vi "Calculate 2D scan positions.vi"(2 "Scan direction":u16(ring) items=["Scan from middle", "Scan upper left", "Scan upper right", "Scan lower left", "Scan lower right", "Scan left", "Scan right", "Scan above", "Scan below"], 3 "Start position ax1":dbl format="%.6f", 4 "Start position ax2":dbl format="%.6f", 6 "Range ax1":dbl format="%.2f", 7 "Step size ax1":dbl format="%.2f", 8 "Range ax2":dbl format="%.2f", 9 "Step size ax2":dbl format="%.2f") -> (10 "Min. pos. ax2":dbl format="%.6f", 11 "Max. pos. ax2":dbl format="%.6f", 12 "1D pos. array ax2":dbl[](array[numeric]) format="%.6f", 13 "No. of steps ax2":i32, 14 "1D pos. array ax1":dbl[](array[numeric]) format="%.6f", 15 "Min. pos. ax1":dbl format="%.6f", 16 "Max. pos. ax1":dbl format="%.6f", 17 "No. of steps ax1":i32, 18 "2D intensity array":dbl[][](array[numeric]) format="%.6f")   [LabVIEW 2020]
doc: "Calculates 2D scan positions according to Scan direction, Start position, Range and Step size of axes 1 and 2 and returns Minimum position, Maximum position, No. of steps and initialized 1D position array for axes 1 and 2 and a 2D intensity array. Scan direction can be \n- Scan from middle meaning that the scan starts at (Start position ax1 - ½ Range ax1, Start position ax2 - ½ Range ax2) and stops at (Start position ax1 + ½ Range ax1, Start position ax2 + ½ Range ax2), \n- Scan upper left meaning that scan starts at (Start position ax1 - Range ax1, Start position ax2) and stops at (Start position ax1, Start position ax2 + Range ax2), \n- Scan upper right meaning that scan starts at (Start position ax1, Start position ax2) and stops at (Start position ax1 + Range ax1, Start position ax2 + Range ax2), \n- Scan lower left meaning that the scan starts at (Start position ax1 - Range ax1, Start position ax2 - Range ax2) and stops at (Start position ax1, Start position ax2), \n- Scan lower right meaning that the scan starts at (Start position ax1, Start position ax2 - Range ax2) and stops at (Start position ax1 + Range ax1, Start position ax2), \n- Scan left meaning that the scan starts at (Start position ax1 - Range ax1, Start position ax2 - ½ Range ax2) and stops at (Start position ax1, Start position ax2 + ½ Range ax2), \n- Scan right meaning that the scan starts at (Start position ax1, Start position ax2 - ½ Range ax2) and stops at (Start position ax1 + Range ax1, Start position ax2 + ½ Range ax2), \n- Scan above meaning that the scan starts at (Start position ax1 - ½ Range ax1, Start position ax2) and stops at (Start position ax1 + ½ Range ax1, Start position ax2 + Range ax2), \n- Scan below meaning that the scan starts at (Start position ax1 - ½ Range ax1, Start position ax2 - Range ax2) and stops at (Start position ax1 + ½ Range ax1, Start position ax2),"
panel:
  # "Calculates 2D scan positions and initialized intensity array."
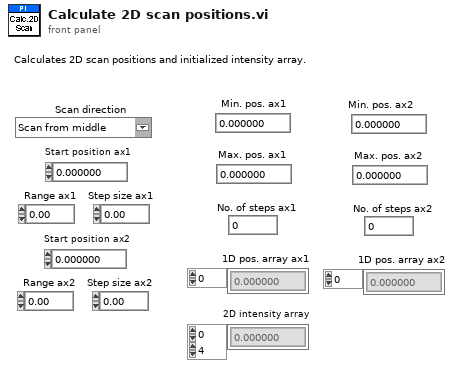
[diagram p1: front panel]
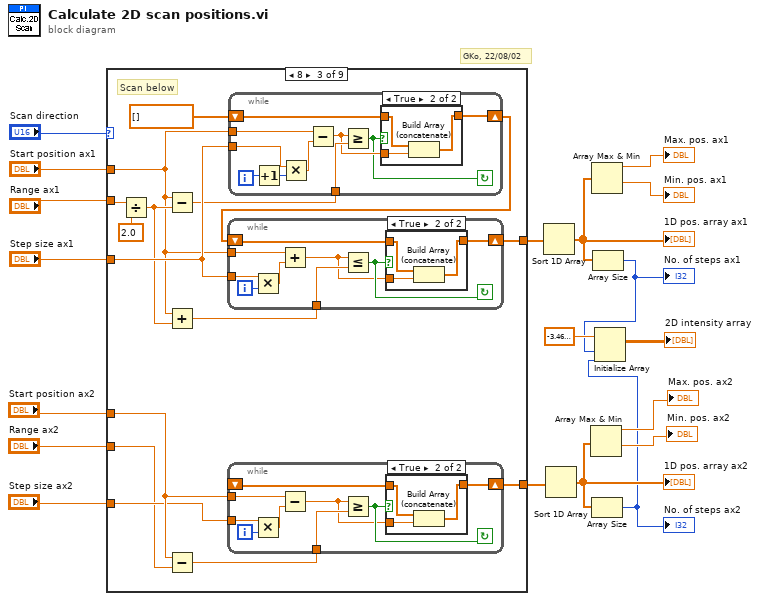
[diagram p0: block diagram]
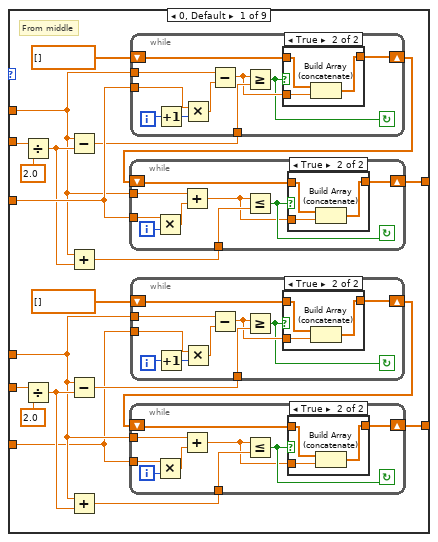
[diagram p2: hidden frame]
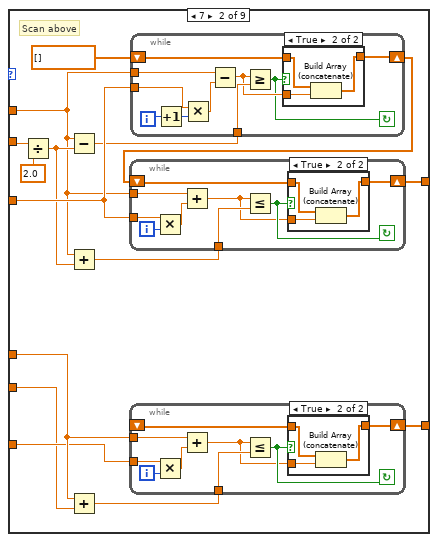
[diagram p7: hidden frame]
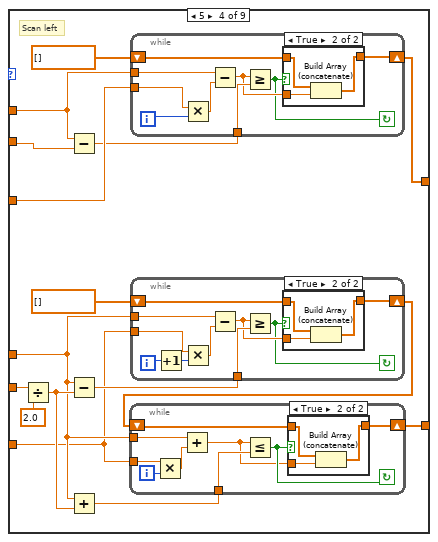
[diagram p14: hidden frame]
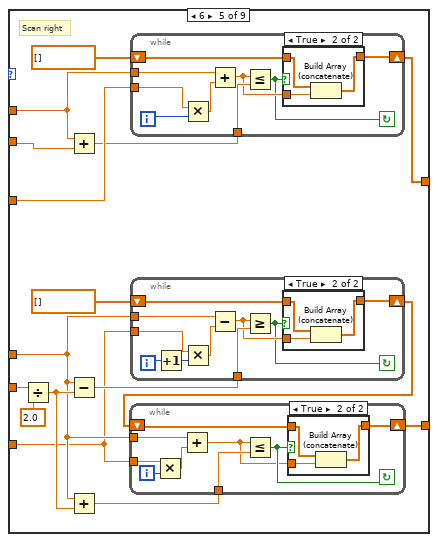
[diagram p18: hidden frame]
diagram:
  # "GKo, 22/08/02"
  n1 = case shown="8" "Scan direction" {
    tunnel: "Range ax1" -> [w39 w108 w163 w204 w260 w325 w363 w401 w439]
    tunnel: "Start position ax1" -> [w34 w103 w158 w218 w274 w326 w364 w402 w440]
    tunnel: "Step size ax1" -> [w36 w105 w160 w219 w275 w327 w365 w403 w441]
    tunnel: [w30 w99 w154 w205 w261 w322 w360 w398 w436] -> w11
    tunnel: [w23 w97 w152 w209 w265 w319 w357 w395 w433] -> w9
    tunnel: "Range ax2" -> [w22 w94 w149 w208 w264 w317 w355 w393 w431]
    tunnel: "Start position ax2" -> [w21 w96 w151 w207 w263 w318 w356 w394 w432]
    tunnel: "Step size ax2" -> [w20 w95 w150 w206 w262 w316 w354 w392 w430]
    frame 0, Default {
      # "From middle"
      n2 = Divide(x=w39, y=2.0) -> (x/y=w35:dbl)
      n3 = Divide(x=w22, y=2.0) -> (x/y=w27:dbl)
      n4 = Subtract(x=w34, y=w35) -> (x-y=w33:dbl)
      n5 = Add(x=w34, y=w35) -> (x+y=w37:dbl)
      n6 = Subtract(x=w21, y=w27) -> (x-y=w26:dbl)
      n7 = Add(x=w21, y=w27) -> (x+y=w28:dbl)
      n8 = while {
        shift-left: dbl[] [] -> [w56]
        shift-right: [w54] -> w31
        tunnel: w33 -> [w57]
        tunnel: w36 -> [w59]
        tunnel: w34 -> [w61]
        i -> [w62]
        stop <- w53 continue-if-true
        n9 = Increment(x=w62) -> (x+1=w60:i32)
        n10 = Multiply(x=w59, y=w60) -> (x*y=w58:dbl)
        n11 = Subtract(x=w61, y=w58) -> (x-y=w55:dbl)
        n12 = Greater Or Equal?(x=w55, y=w57) -> (x >= y?=w53:bool)
        n13 = case shown="True" w53 {
          tunnel: [w63 w66] -> w54
          tunnel: w56 -> [w63 w65]
          tunnel: w55 -> [_ w64]
          frame False {
          }
          frame True {
            n14 = Build Array (concatenate)(w65, w64) -> (w66:dbl[])
          }
        }
      }
      n15 = while {
        tunnel: w37 -> [w42]
        shift-left: w31 -> [w43]
        shift-right: [w44] -> w30
        tunnel: w34 -> [w46]
        tunnel: w36 -> [w47]
        i -> [w48]
        stop <- w41 continue-if-true
        n16 = Multiply(x=w47, y=w48) -> (x*y=w45:dbl)
        n17 = Add(x=w46, y=w45) -> (x+y=w40:dbl)
        n18 = Less Or Equal?(x=w40, y=w42) -> (x <= y?=w41:bool)
        n19 = case shown="True" w41 {
          tunnel: [w49 w52] -> w44
          tunnel: w43 -> [w49 w51]
          tunnel: w40 -> [_ w50]
          frame False {
          }
          frame True {
            n20 = Build Array (concatenate)(w51, w50) -> (w52:dbl[])
          }
        }
      }
      n21 = while {
        shift-left: dbl[] [] -> [w83]
        shift-right: [w81] -> w24
        tunnel: w26 -> [w84]
        tunnel: w20 -> [w86]
        tunnel: w21 -> [w88]
        i -> [w89]
        stop <- w80 continue-if-true
        n22 = Increment(x=w89) -> (x+1=w87:i32)
        n23 = Multiply(x=w86, y=w87) -> (x*y=w85:dbl)
        n24 = Subtract(x=w88, y=w85) -> (x-y=w82:dbl)
        n25 = Greater Or Equal?(x=w82, y=w84) -> (x >= y?=w80:bool)
        n26 = case shown="True" w80 {
          tunnel: [w90 w93] -> w81
          tunnel: w83 -> [w90 w92]
          tunnel: w82 -> [_ w91]
          frame False {
          }
          frame True {
            n27 = Build Array (concatenate)(w92, w91) -> (w93:dbl[])
          }
        }
      }
      n28 = while {
        tunnel: w28 -> [w69]
        shift-left: w24 -> [w70]
        shift-right: [w71] -> w23
        tunnel: w21 -> [w73]
        tunnel: w20 -> [w74]
        i -> [w75]
        stop <- w68 continue-if-true
        n29 = Multiply(x=w74, y=w75) -> (x*y=w72:dbl)
        n30 = Add(x=w73, y=w72) -> (x+y=w67:dbl)
        n31 = Less Or Equal?(x=w67, y=w69) -> (x <= y?=w68:bool)
        n32 = case shown="True" w68 {
          tunnel: [w76 w79] -> w71
          tunnel: w70 -> [w76 w78]
          tunnel: w67 -> [_ w77]
          frame False {
          }
          frame True {
            n33 = Build Array (concatenate)(w78, w77) -> (w79:dbl[])
          }
        }
      }
    }
    frame 7 {
      # "Scan above"
      n34 = Divide(x=w108, y=2.0) -> (x/y=w104:dbl)
      n35 = Subtract(x=w103, y=w104) -> (x-y=w102:dbl)
      n36 = Add(x=w103, y=w104) -> (x+y=w106:dbl)
      n37 = Add(x=w96, y=w94) -> (x+y=w98:dbl)
      n38 = while {
        tunnel: w98 -> [w138]
        shift-left: _ -> [w139]
        shift-right: [w140] -> w97
        tunnel: w96 -> [w142]
        tunnel: w95 -> [w143]
        i -> [w144]
        stop <- w137 continue-if-true
        n39 = Multiply(x=w143, y=w144) -> (x*y=w141:dbl)
        n40 = Add(x=w142, y=w141) -> (x+y=w136:dbl)
        n41 = Less Or Equal?(x=w136, y=w138) -> (x <= y?=w137:bool)
        n42 = case shown="True" w137 {
          tunnel: [w145 w148] -> w140
          tunnel: w139 -> [w145 w147]
          tunnel: w136 -> [_ w146]
          frame False {
          }
          frame True {
            n43 = Build Array (concatenate)(w147, w146) -> (w148:dbl[])
          }
        }
      }
      n44 = while {
        shift-left: dbl[] [] -> [w125]
        shift-right: [w123] -> w100
        tunnel: w102 -> [w126]
        tunnel: w105 -> [w128]
        tunnel: w103 -> [w130]
        i -> [w131]
        stop <- w122 continue-if-true
        n45 = Increment(x=w131) -> (x+1=w129:i32)
        n46 = Multiply(x=w128, y=w129) -> (x*y=w127:dbl)
        n47 = Subtract(x=w130, y=w127) -> (x-y=w124:dbl)
        n48 = Greater Or Equal?(x=w124, y=w126) -> (x >= y?=w122:bool)
        n49 = case shown="True" w122 {
          tunnel: [w132 w135] -> w123
          tunnel: w125 -> [w132 w134]
          tunnel: w124 -> [_ w133]
          frame False {
          }
          frame True {
            n50 = Build Array (concatenate)(w134, w133) -> (w135:dbl[])
          }
        }
      }
      n51 = while {
        tunnel: w106 -> [w111]
        shift-left: w100 -> [w112]
        shift-right: [w113] -> w99
        tunnel: w103 -> [w115]
        tunnel: w105 -> [w116]
        i -> [w117]
        stop <- w110 continue-if-true
        n52 = Multiply(x=w116, y=w117) -> (x*y=w114:dbl)
        n53 = Add(x=w115, y=w114) -> (x+y=w109:dbl)
        n54 = Less Or Equal?(x=w109, y=w111) -> (x <= y?=w110:bool)
        n55 = case shown="True" w110 {
          tunnel: [w118 w121] -> w113
          tunnel: w112 -> [w118 w120]
          tunnel: w109 -> [_ w119]
          frame False {
          }
          frame True {
            n56 = Build Array (concatenate)(w120, w119) -> (w121:dbl[])
          }
        }
      }
    }
    frame 8 {
      # "Scan below"
      n57 = Divide(x=w163, y=2.0) -> (x/y=w159:dbl)
      n58 = Subtract(x=w158, y=w159) -> (x-y=w157:dbl)
      n59 = Add(x=w158, y=w159) -> (x+y=w161:dbl)
      n60 = Subtract(x=w151, y=w149) -> (x-y=w153:dbl)
      n61 = while {
        tunnel: w153 -> [w193]
        shift-left: _ -> [w194]
        shift-right: [w195] -> w152
        tunnel: w151 -> [w197]
        tunnel: w150 -> [w198]
        i -> [w199]
        stop <- w192 continue-if-true
        n62 = Multiply(x=w198, y=w199) -> (x*y=w196:dbl)
        n63 = Subtract(x=w197, y=w196) -> (x-y=w191:dbl)
        n64 = Greater Or Equal?(x=w191, y=w193) -> (x >= y?=w192:bool)
        n65 = case shown="True" w192 {
          tunnel: [w200 w203] -> w195
          tunnel: w194 -> [w200 w202]
          tunnel: w191 -> [_ w201]
          frame False {
          }
          frame True {
            n66 = Build Array (concatenate)(w202, w201) -> (w203:dbl[])
          }
        }
      }
      n67 = while {
        shift-left: dbl[] [] -> [w180]
        shift-right: [w178] -> w155
        tunnel: w157 -> [w181]
        tunnel: w160 -> [w183]
        tunnel: w158 -> [w185]
        i -> [w186]
        stop <- w177 continue-if-true
        n68 = Increment(x=w186) -> (x+1=w184:i32)
        n69 = Multiply(x=w183, y=w184) -> (x*y=w182:dbl)
        n70 = Subtract(x=w185, y=w182) -> (x-y=w179:dbl)
        n71 = Greater Or Equal?(x=w179, y=w181) -> (x >= y?=w177:bool)
        n72 = case shown="True" w177 {
          tunnel: [w187 w190] -> w178
          tunnel: w180 -> [w187 w189]
          tunnel: w179 -> [_ w188]
          frame False {
          }
          frame True {
            n73 = Build Array (concatenate)(w189, w188) -> (w190:dbl[])
          }
        }
      }
      n74 = while {
        tunnel: w161 -> [w166]
        shift-left: w155 -> [w167]
        shift-right: [w168] -> w154
        tunnel: w158 -> [w170]
        tunnel: w160 -> [w171]
        i -> [w172]
        stop <- w165 continue-if-true
        n75 = Multiply(x=w171, y=w172) -> (x*y=w169:dbl)
        n76 = Add(x=w170, y=w169) -> (x+y=w164:dbl)
        n77 = Less Or Equal?(x=w164, y=w166) -> (x <= y?=w165:bool)
        n78 = case shown="True" w165 {
          tunnel: [w173 w176] -> w168
          tunnel: w167 -> [w173 w175]
          tunnel: w164 -> [_ w174]
          frame False {
          }
          frame True {
            n79 = Build Array (concatenate)(w175, w174) -> (w176:dbl[])
          }
        }
      }
    }
    frame 5 {
      # "Scan left"
      n80 = Divide(x=w208, y=2.0) -> (x/y=w213:dbl)
      n81 = Subtract(x=w218, y=w204) -> (x-y=w217:dbl)
      n82 = Subtract(x=w207, y=w213) -> (x-y=w212:dbl)
      n83 = Add(x=w207, y=w213) -> (x+y=w214:dbl)
      n84 = while {
        shift-left: dbl[] [] -> [w224]
        shift-right: [w222] -> w205
        tunnel: w217 -> [w225]
        tunnel: w219 -> [w227]
        tunnel: w218 -> [w228]
        i -> [w220]
        stop <- w221 continue-if-true
        n85 = Multiply(x=w227, y=w220) -> (x*y=w226:dbl)
        n86 = Subtract(x=w228, y=w226) -> (x-y=w223:dbl)
        n87 = Greater Or Equal?(x=w223, y=w225) -> (x >= y?=w221:bool)
        n88 = case shown="True" w221 {
          tunnel: [w229 w232] -> w222
          tunnel: w224 -> [w229 w231]
          tunnel: w223 -> [_ w230]
          frame False {
          }
          frame True {
            n89 = Build Array (concatenate)(w231, w230) -> (w232:dbl[])
          }
        }
      }
      n90 = while {
        shift-left: dbl[] [] -> [w249]
        shift-right: [w247] -> w210
        tunnel: w212 -> [w250]
        tunnel: w206 -> [w252]
        tunnel: w207 -> [w254]
        i -> [w255]
        stop <- w246 continue-if-true
        n91 = Increment(x=w255) -> (x+1=w253:i32)
        n92 = Multiply(x=w252, y=w253) -> (x*y=w251:dbl)
        n93 = Subtract(x=w254, y=w251) -> (x-y=w248:dbl)
        n94 = Greater Or Equal?(x=w248, y=w250) -> (x >= y?=w246:bool)
        n95 = case shown="True" w246 {
          tunnel: [w256 w259] -> w247
          tunnel: w249 -> [w256 w258]
          tunnel: w248 -> [_ w257]
          frame False {
          }
          frame True {
            n96 = Build Array (concatenate)(w258, w257) -> (w259:dbl[])
          }
        }
      }
      n97 = while {
        tunnel: w214 -> [w235]
        shift-left: w210 -> [w236]
        shift-right: [w237] -> w209
        tunnel: w207 -> [w239]
        tunnel: w206 -> [w240]
        i -> [w241]
        stop <- w234 continue-if-true
        n98 = Multiply(x=w240, y=w241) -> (x*y=w238:dbl)
        n99 = Add(x=w239, y=w238) -> (x+y=w233:dbl)
        n100 = Less Or Equal?(x=w233, y=w235) -> (x <= y?=w234:bool)
        n101 = case shown="True" w234 {
          tunnel: [w242 w245] -> w237
          tunnel: w236 -> [w242 w244]
          tunnel: w233 -> [_ w243]
          frame False {
          }
          frame True {
            n102 = Build Array (concatenate)(w244, w243) -> (w245:dbl[])
          }
        }
      }
    }
    frame 6 {
      # "Scan right"
      n103 = Divide(x=w264, y=2.0) -> (x/y=w269:dbl)
      n104 = Add(x=w274, y=w260) -> (x+y=w273:dbl)
      n105 = Subtract(x=w263, y=w269) -> (x-y=w268:dbl)
      n106 = Add(x=w263, y=w269) -> (x+y=w270:dbl)
      n107 = while {
        shift-left: dbl[] [] -> [w280]
        shift-right: [w278] -> w261
        tunnel: w273 -> [w281]
        tunnel: w275 -> [w283]
        tunnel: w274 -> [w284]
        i -> [w276]
        stop <- w277 continue-if-true
        n108 = Multiply(x=w283, y=w276) -> (x*y=w282:dbl)
        n109 = Add(x=w284, y=w282) -> (x+y=w279:dbl)
        n110 = Less Or Equal?(x=w279, y=w281) -> (x <= y?=w277:bool)
        n111 = case shown="True" w277 {
          tunnel: [w285 w288] -> w278
          tunnel: w280 -> [w285 w287]
          tunnel: w279 -> [_ w286]
          frame False {
          }
          frame True {
            n112 = Build Array (concatenate)(w287, w286) -> (w288:dbl[])
          }
        }
      }
      n113 = while {
        shift-left: dbl[] [] -> [w305]
        shift-right: [w303] -> w266
        tunnel: w268 -> [w306]
        tunnel: w262 -> [w308]
        tunnel: w263 -> [w310]
        i -> [w311]
        stop <- w302 continue-if-true
        n114 = Increment(x=w311) -> (x+1=w309:i32)
        n115 = Multiply(x=w308, y=w309) -> (x*y=w307:dbl)
        n116 = Subtract(x=w310, y=w307) -> (x-y=w304:dbl)
        n117 = Greater Or Equal?(x=w304, y=w306) -> (x >= y?=w302:bool)
        n118 = case shown="True" w302 {
          tunnel: [w312 w315] -> w303
          tunnel: w305 -> [w312 w314]
          tunnel: w304 -> [_ w313]
          frame False {
          }
          frame True {
            n119 = Build Array (concatenate)(w314, w313) -> (w315:dbl[])
          }
        }
      }
      n120 = while {
        tunnel: w270 -> [w291]
        shift-left: w266 -> [w292]
        shift-right: [w293] -> w265
        tunnel: w263 -> [w295]
        tunnel: w262 -> [w296]
        i -> [w297]
        stop <- w290 continue-if-true
        n121 = Multiply(x=w296, y=w297) -> (x*y=w294:dbl)
        n122 = Add(x=w295, y=w294) -> (x+y=w289:dbl)
        n123 = Less Or Equal?(x=w289, y=w291) -> (x <= y?=w290:bool)
        n124 = case shown="True" w290 {
          tunnel: [w298 w301] -> w293
          tunnel: w292 -> [w298 w300]
          tunnel: w289 -> [_ w299]
          frame False {
          }
          frame True {
            n125 = Build Array (concatenate)(w300, w299) -> (w301:dbl[])
          }
        }
      }
    }
    frame 1 {
      # "Scan upper left"
      n126 = Subtract(x=w326, y=w325) -> (x-y=w324:dbl)
      n127 = Add(x=w318, y=w317) -> (x+y=w321:dbl)
      n128 = while {
        tunnel: w324 -> [w328]
        shift-left: dbl[] [] -> [w332]
        shift-right: [w331] -> w322
        tunnel: w327 -> [w334]
        tunnel: w326 -> [w336]
        i -> [w335]
        stop <- w330 continue-if-true
        n129 = Multiply(x=w334, y=w335) -> (x*y=w333:dbl)
        n130 = Subtract(x=w336, y=w333) -> (x-y=w329:dbl)
        n131 = Greater Or Equal?(x=w329, y=w328) -> (x >= y?=w330:bool)
        n132 = case shown="True" w330 {
          tunnel: [w337 w340] -> w331
          tunnel: w332 -> [w337 w339]
          tunnel: w329 -> [_ w338]
          frame False {
          }
          frame True {
            n133 = Build Array (concatenate)(w339, w338) -> (w340:dbl[])
          }
        }
      }
      n134 = while {
        tunnel: w321 -> [w341]
        shift-left: dbl[] [] -> [w345]
        shift-right: [w344] -> w319
        tunnel: w316 -> [w347]
        tunnel: w318 -> [w349]
        i -> [w348]
        stop <- w343 continue-if-true
        n135 = Multiply(x=w347, y=w348) -> (x*y=w346:dbl)
        n136 = Add(x=w349, y=w346) -> (x+y=w342:dbl)
        n137 = Less Or Equal?(x=w342, y=w341) -> (x <= y?=w343:bool)
        n138 = case shown="True" w343 {
          tunnel: [w350 w353] -> w344
          tunnel: w345 -> [w350 w352]
          tunnel: w342 -> [_ w351]
          frame False {
          }
          frame True {
            n139 = Build Array (concatenate)(w352, w351) -> (w353:dbl[])
          }
        }
      }
    }
    frame 2 {
      # "Scan upper right"
      n140 = Add(x=w364, y=w363) -> (x+y=w362:dbl)
      n141 = Add(x=w356, y=w355) -> (x+y=w359:dbl)
      n142 = while {
        tunnel: w362 -> [w366]
        shift-left: dbl[] [] -> [w370]
        shift-right: [w369] -> w360
        tunnel: w365 -> [w372]
        tunnel: w364 -> [w374]
        i -> [w373]
        stop <- w368 continue-if-true
        n143 = Multiply(x=w372, y=w373) -> (x*y=w371:dbl)
        n144 = Add(x=w374, y=w371) -> (x+y=w367:dbl)
        n145 = Less Or Equal?(x=w367, y=w366) -> (x <= y?=w368:bool)
        n146 = case shown="True" w368 {
          tunnel: [w375 w378] -> w369
          tunnel: w370 -> [w375 w377]
          tunnel: w367 -> [_ w376]
          frame False {
          }
          frame True {
            n147 = Build Array (concatenate)(w377, w376) -> (w378:dbl[])
          }
        }
      }
      n148 = while {
        tunnel: w359 -> [w379]
        shift-left: dbl[] [] -> [w383]
        shift-right: [w382] -> w357
        tunnel: w354 -> [w385]
        tunnel: w356 -> [w387]
        i -> [w386]
        stop <- w381 continue-if-true
        n149 = Multiply(x=w385, y=w386) -> (x*y=w384:dbl)
        n150 = Add(x=w387, y=w384) -> (x+y=w380:dbl)
        n151 = Less Or Equal?(x=w380, y=w379) -> (x <= y?=w381:bool)
        n152 = case shown="True" w381 {
          tunnel: [w388 w391] -> w382
          tunnel: w383 -> [w388 w390]
          tunnel: w380 -> [_ w389]
          frame False {
          }
          frame True {
            n153 = Build Array (concatenate)(w390, w389) -> (w391:dbl[])
          }
        }
      }
    }
    frame 3 {
      # "Scan lower left"
      n154 = Subtract(x=w402, y=w401) -> (x-y=w400:dbl)
      n155 = Subtract(x=w394, y=w393) -> (x-y=w397:dbl)
      n156 = while {
        tunnel: w400 -> [w404]
        shift-left: dbl[] [] -> [w408]
        shift-right: [w407] -> w398
        tunnel: w403 -> [w410]
        tunnel: w402 -> [w412]
        i -> [w411]
        stop <- w406 continue-if-true
        n157 = Multiply(x=w410, y=w411) -> (x*y=w409:dbl)
        n158 = Subtract(x=w412, y=w409) -> (x-y=w405:dbl)
        n159 = Greater Or Equal?(x=w405, y=w404) -> (x >= y?=w406:bool)
        n160 = case shown="True" w406 {
          tunnel: [w413 w416] -> w407
          tunnel: w408 -> [w413 w415]
          tunnel: w405 -> [_ w414]
          frame False {
          }
          frame True {
            n161 = Build Array (concatenate)(w415, w414) -> (w416:dbl[])
          }
        }
      }
      n162 = while {
        tunnel: w397 -> [w417]
        shift-left: dbl[] [] -> [w421]
        shift-right: [w420] -> w395
        tunnel: w392 -> [w423]
        tunnel: w394 -> [w425]
        i -> [w424]
        stop <- w419 continue-if-true
        n163 = Multiply(x=w423, y=w424) -> (x*y=w422:dbl)
        n164 = Subtract(x=w425, y=w422) -> (x-y=w418:dbl)
        n165 = Greater Or Equal?(x=w418, y=w417) -> (x >= y?=w419:bool)
        n166 = case shown="True" w419 {
          tunnel: [w426 w429] -> w420
          tunnel: w421 -> [w426 w428]
          tunnel: w418 -> [_ w427]
          frame False {
          }
          frame True {
            n167 = Build Array (concatenate)(w428, w427) -> (w429:dbl[])
          }
        }
      }
    }
    frame 4 {
      # "Scan lower right"
      n168 = Add(x=w440, y=w439) -> (x+y=w438:dbl)
      n169 = Subtract(x=w432, y=w431) -> (x-y=w435:dbl)
      n170 = while {
        tunnel: w438 -> [w442]
        shift-left: dbl[] [] -> [w446]
        shift-right: [w445] -> w436
        tunnel: w441 -> [w448]
        tunnel: w440 -> [w450]
        i -> [w449]
        stop <- w444 continue-if-true
        n171 = Multiply(x=w448, y=w449) -> (x*y=w447:dbl)
        n172 = Add(x=w450, y=w447) -> (x+y=w443:dbl)
        n173 = Less Or Equal?(x=w443, y=w442) -> (x <= y?=w444:bool)
        n174 = case shown="True" w444 {
          tunnel: [w451 w454] -> w445
          tunnel: w446 -> [w451 w453]
          tunnel: w443 -> [_ w452]
          frame False {
          }
          frame True {
            n175 = Build Array (concatenate)(w453, w452) -> (w454:dbl[])
          }
        }
      }
      n176 = while {
        tunnel: w435 -> [w455]
        shift-left: dbl[] [] -> [w459]
        shift-right: [w458] -> w433
        tunnel: w430 -> [w461]
        tunnel: w432 -> [w463]
        i -> [w462]
        stop <- w457 continue-if-true
        n177 = Multiply(x=w461, y=w462) -> (x*y=w460:dbl)
        n178 = Subtract(x=w463, y=w460) -> (x-y=w456:dbl)
        n179 = Greater Or Equal?(x=w456, y=w455) -> (x >= y?=w457:bool)
        n180 = case shown="True" w457 {
          tunnel: [w464 w467] -> w458
          tunnel: w459 -> [w464 w466]
          tunnel: w456 -> [_ w465]
          frame False {
          }
          frame True {
            n181 = Build Array (concatenate)(w466, w465) -> (w467:dbl[])
          }
        }
      }
    }
  }
  n182 = Sort 1D Array(array=w11) -> (sorted array=w13:dbl[])
  "1D pos. array ax1" <- w13
  n183 = Sort 1D Array(array=w9) -> (sorted array=w6:dbl[])
  "1D pos. array ax2" <- w6
  n184 = Array Max & Min(array=w6) -> (max value=→"Max. pos. ax2":dbl, min value=→"Min. pos. ax2":dbl)  [unwired: 2 out]
  n185 = Array Max & Min(array=w13) -> (max value=→"Max. pos. ax1":dbl, min value=→"Min. pos. ax1":dbl)  [unwired: 2 out]
  n186 = Array Size(array=w6) -> (size(s)=w1:i32)
  "No. of steps ax2" <- w1
  n187 = Array Size(array=w13) -> (size(s)=w2:i32)
  "No. of steps ax1" <- w2
  n188 = Initialize Array(-3.469446951953614e-18 ("Element Data"), w2, w1) -> (→"2D intensity array":dbl[][])
